vi "OffsetRect by HV and Rect.vi"(8 "错误输入":errorcluster, 9 "v":i16, 10 "h":i16, 11 "rect":T1 caption="矩形") -> (0 "错误输出":errorcluster, 3 "offset rect":T1 caption="偏移矩形")   [LabVIEW 2012, in "Rect Tools.lvlib"]
uses:
  Rect Tools.lvlib
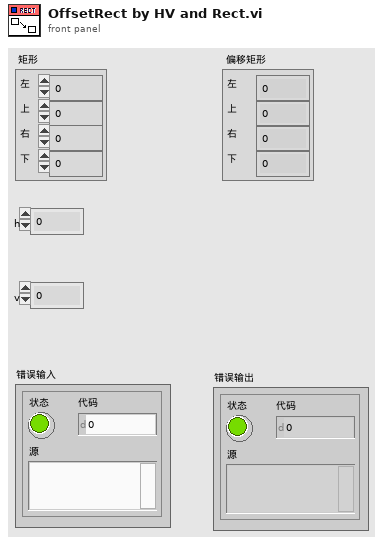
[diagram p1: front panel]
types:
  T1 = cluster{"left":i16, "top":i16, "right":i16, "bottom":i16}
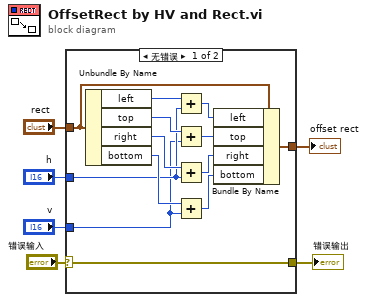
[diagram p0: block diagram]
diagram:
  n1 = case shown="无错误" "错误输入" {
    selector: "错误输入" -> [w11 w21]
    tunnel: [w11 w21] -> w5
    tunnel: "rect" -> [w10 w20]
    tunnel: [w9 w20] -> w3
    tunnel: "h" -> [w8 _]
    tunnel: "v" -> [w7 _]
    frame No Error {
      n2 = Unbundle By Name(w10) -> ("left"=w18:i16, "top"=w17:i16, "right"=w16:i16, "bottom"=w15:i16)
      n3 = Add(x=w18, y=w8) -> (x+y=w19:i16)
      n4 = Add(x=w17, y=w7) -> (x+y=w12:i16)
      n5 = Add(x=w16, y=w8) -> (x+y=w13:i16)
      n6 = Add(x=w15, y=w7) -> (x+y=w14:i16)
      n7 = Bundle By Name(cluster=w10, "left"=w19, "top"=w12, "right"=w13, "bottom"=w14) -> (w9:T1)
    }
    frame Error {
    }
  }
  "错误输出" <- w5
  "offset rect" <- w3
